vi "print_llm_response.vi"(8 "error in (no error)":errorcluster, 10 "llm_response":refnum<class "abstract_message_base.lvclass">, 11 "simple_html_chat_ui in":refnum<class "simple_html_chat_ui.lvclass">) -> (0 "error out":errorcluster, 3 "simple_html_chat_ui out":refnum<class "simple_html_chat_ui.lvclass">)   [LabVIEW 2020, in "simple_html_chat_ui.lvclass"]
uses:
  simple_html_chat_ui.lvclass
  models/abstract_message_base/abstract_message_base.lvclass
  models/message_text/message_text.lvclass
  simple_html_chat_ui.lvclass/simple_html_chat_ui.ctl
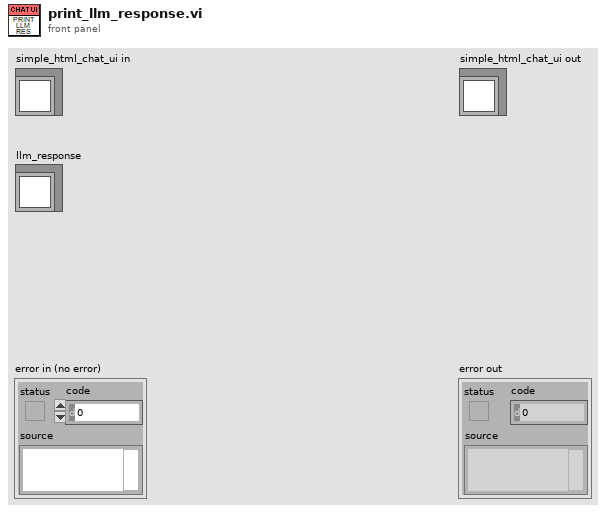
[diagram p1: front panel]
types:
  T1 = typedef "message_text.lvclass/message.ctl" = cluster{"role":string, "content":string[]}
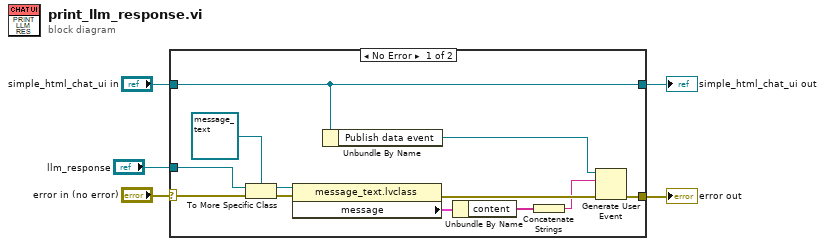
[diagram p0: block diagram]
diagram:
  n1 = case shown="No Error" "error in (no error)" {
    selector: "error in (no error)" -> [w14 w19]
    tunnel: [w10 w19] -> w4
    tunnel: [w12 w18] -> w2
    tunnel: "simple_html_chat_ui in" -> [w12 w18]
    tunnel: "llm_response" -> [w13 _]
    frame No Error {
      n2 = To More Specific Class(target class=refnum<class "message_text.lvclass"> refnum ("message_text.lvclass"), reference=w13, error in=w14) -> (specific class reference=w16:refnum<class "message_text.lvclass">, error out=w15:errorcluster)
      n3 = property class="message_text.lvclass"(reference=w16, error in=w15) -> (error out=w11:errorcluster, "message"=w7:T1)  [unwired: 1 out]
      n4 = Unbundle By Name(w12) -> ("Publish data event"=w9:refnum<user-event>)
      n5 = Unbundle By Name(w7) -> ("content"=w8:string[])
      n6 = Concatenate Strings(w8) -> (w6:string)
      n7 = Generate User Event(user event=w9, event data cluster=w6, error in=w11) -> (error out=w10:errorcluster)  [unwired: 1 in, 1 out]
    }
    frame Error {
    }
  }
  "error out" <- w4
  "simple_html_chat_ui out" <- w2
